vi "init.vi"(8 "error in":errorcluster, 10 "TBM module configuration in":refnum<class "TBM module configuration.lvclass">, 11 "Polynomial Scale runtime in":refnum<class "Polynomial Scale runtime.lvclass">) -> (0 "error out":errorcluster, 1 "data allocations":T1, 2 "execution settings":T4, 3 "Polynomial Scale runtime out":refnum<class "Polynomial Scale runtime.lvclass">)   [LabVIEW 2013, in "Polynomial Scale runtime.lvclass"]
doc: "Provides an interface for initializing a module at runtime. While this interface performs no operations, a child should provide an override which may open any necessary references or sessions, allocate necessary memory, and perform any final configuration validataion before providing the full configuration <b>execution data</b> to the calling process."
uses:
  Polynomial Scale runtime.lvclass
  <vilib>/NI/Tag Bus Module Framework/module configuration/TBM module configuration.lvclass
  <vilib>/NI/Tag Bus Module Framework/runtime/execution settings.ctl
  <vilib>/NI/Tag Bus Module Framework/channel/data tables.ctl
  <vilib>/NI/Tag Bus/dictionary/data dictionary.lvclass
  <vilib>/NI/Tag Bus/dictionary table pair.ctl
  <vilib>/NI/Tag Bus/table/data table.ctl
  configuration/Polynomial Scale configuration.lvclass
  <vilib>/NI/DCAF Templates/DCAF Scaling/module/execution/Scaling runtime.lvclass
  configuration/Polynomial Scale configuration.lvclass/Polynomial Scale configuration.ctl
  Polynomial Scale runtime.lvclass/Polynomial Scale runtime.ctl
  <vilib>/NI/Tag Bus Module Framework/channel/TBM channel.lvclass
  <vilib>/NI/Tag Bus Module Framework/runtime/TBM module execution interface.lvclass
  <vilib>/NI/Tag Bus/tag bus.lvlib
  <vilib>/NI/Tag Bus/table/data table.lvlib
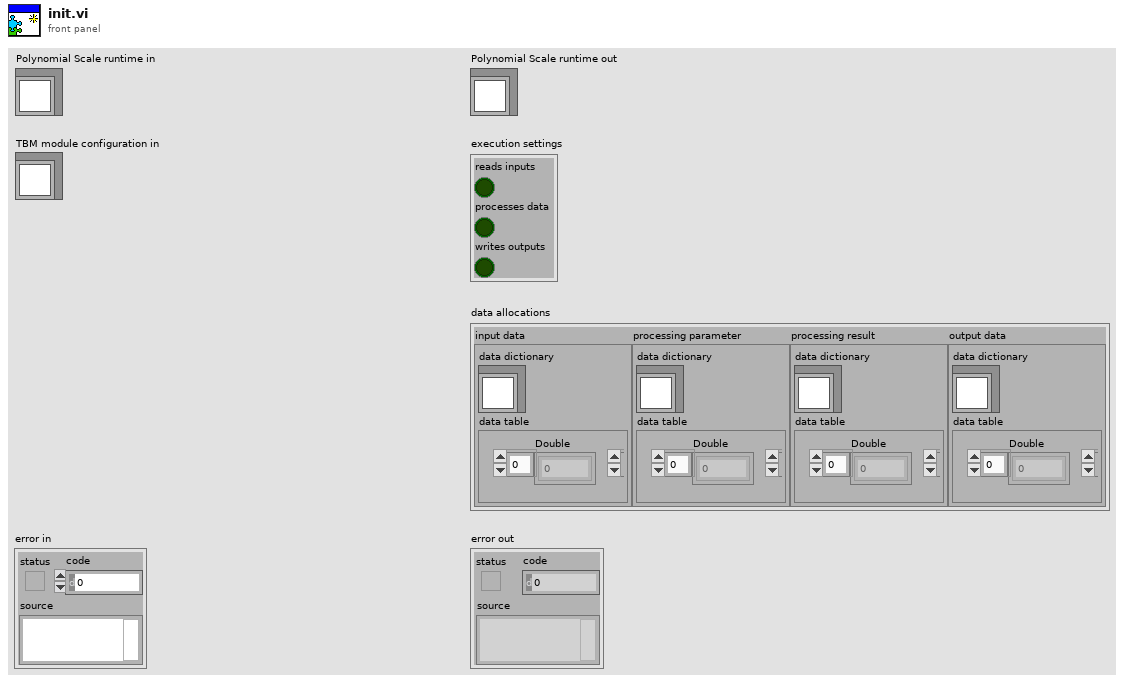
[diagram p1: front panel]
types:
  T1 = typedef "TBM channel.lvclass/data tables.ctl" = cluster{"input data":T2, "processing parameter":T2, "processing result":T2, "output data":T2}
  T2 = typedef "tag bus.lvlib/dictionary table pair.ctl" = cluster{"data dictionary":refnum<class "data dictionary.lvclass">, "data table":T3}
  T3 = typedef "tag bus.lvlib/data table.lvlib/data table.ctl" = cluster{"Double":dbl[], "Single":sgl[], "I64":i64[], "I32":i32[], "I16":i16[], "I8":i8[], "U64":u64[], "U32":u32[], "U16":u16[], "U8":u8[], "Boolean":bool[], "String":string[], "Array of Double":cluster{"DBL Array":dbl[]}[], "Array of Single":cluster{"SGL Array":sgl[]}[], "Array of I64":cluster{"I64 Array":i64[]}[], "Array of I32":cluster{"I32 Array":i32[]}[], "Array of I16":cluster{"I16 Array":i16[]}[], "Array of I8":cluster{"I8 Array":i8[]}[], "Array of U64":cluster{"U64 Array":u64[]}[], "Array of U32":cluster{"U32 Array":u32[]}[], "Array of U16":cluster{"U16 Array":u16[]}[], "Array of U8":cluster{"U8 Array":u8[]}[], "Array of Boolean":cluster{"Boolean Array":bool[]}[], "Array of String":cluster{"String Array":string[]}[]}
  T4 = typedef "TBM module execution interface.lvclass/execution settings.ctl" = cluster{"reads inputs":bool, "processes data":bool, "writes outputs":bool}
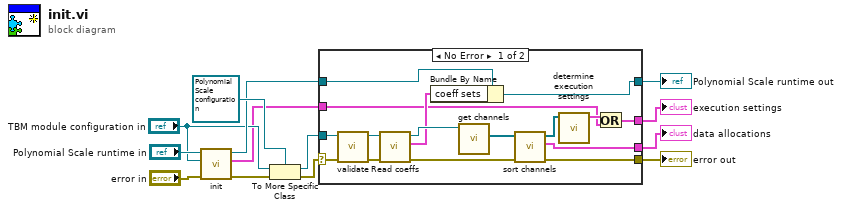
[diagram p0: block diagram]
diagram:
  n1 = call-parent "init.vi"("error in"="error in", "TBM module configuration in"="TBM module configuration in", "Scaling runtime in"="Polynomial Scale runtime in") -> ("error out"=w5:errorcluster, "execution settings"=w1:T4, "Scaling runtime out"=w3:refnum<class "Polynomial Scale runtime.lvclass">)  [unwired: 5 in, 1 out]
  n2 = To More Specific Class(target class=refnum<class "Polynomial Scale configuration.lvclass"> refnum ("Synchronous module configuration"), reference="TBM module configuration in", error in=w5) -> (specific class reference=w12:refnum<class "Polynomial Scale configuration.lvclass">, error out=w13:errorcluster)
  n3 = case shown="No Error" w13 {
    selector: w13 -> [w26 w30]
    tunnel: w12 -> [w25 _]
    tunnel: w3 -> [w19 w31]
    tunnel: [w17 w31] -> w10
    tunnel: [w29 w30] -> w9
    tunnel: [w27 _] -> w7
    tunnel: [w14 _] -> w8
    tunnel: w1 -> [w15 _]
    frame No Error {
      n4 = call-dynamic "validate.vi"("error in"=w26, "Polynomial Scale configuration in"=w25) -> ("error out"=w21:errorcluster, "Polynomial Scale configuration out"=w23:refnum<class "Polynomial Scale configuration.lvclass">)  [unwired: 8 in]
      n5 = call "Read coeffs.vi"("error in (no error)"=w21, "Polynomial Scale configuration in"=w23) -> ("error out"=w20:errorcluster, "coeff sets"=w18:cluster{"coeffs":dbl[]}[], "Polynomial Scale configuration out"=w22:refnum<class "Polynomial Scale configuration.lvclass">)  [unwired: 7 in]
      n6 = Bundle By Name(cluster=w19, "coeff sets"=w18) -> (w17:refnum<class "Polynomial Scale runtime.lvclass">)
      n7 = call-dynamic "get channels.vi"("Scaling configuration in"=w22) -> ("channels"=w24:refnum<class "TBM channel.lvclass">[])  [unwired: 9 in, 1 out]
      n8 = call <vilib>:"sort channels.vi"("error in"=w20, "channels in"=w24) -> ("error out"=w29:errorcluster, "data allocations"=w27:T1, "channels out"=w28:refnum<class "TBM channel.lvclass">[])  [unwired: 7 in]
      n9 = call <vilib>:"determine execution settings.vi"("channels"=w28) -> ("execution settings"=w16:T4)  [unwired: 10 in]
      n10 = Or(x=w16, y=w15) -> (x .or. y?=w14:T4)
    }
    frame Error {
    }
  }
  "error out" <- w9
  "Polynomial Scale runtime out" <- w10
  "execution settings" <- w8
  "data allocations" <- w7
